vi "Configure Maker Units.vi"(6 "Reset Y Position (T: Enable)":bool=TRUE, 7 "Reset X Position (T: Enable)":bool=TRUE, 8 "error in (no error)":errorcluster, 9 "Marker Y Units (0: Base)":i32(ring) items=["Base", "Percent"], 10 "Marker X Units (0: Seconds)":i32(ring) items=["Seconds", "Hertz", "Degrees", "Percent"], 11 "VISA resource name":refnum<visa-resource-name>) -> (0 "error out":errorcluster, 3 "VISA resource name out":refnum<visa-resource-name>)   [LabVIEW 2016, in "Agilent 2000 3000 X-Series.lvlib"]
doc: "Configures the marker unit settings."
uses:
  Agilent 2000 3000 X-Series.lvlib
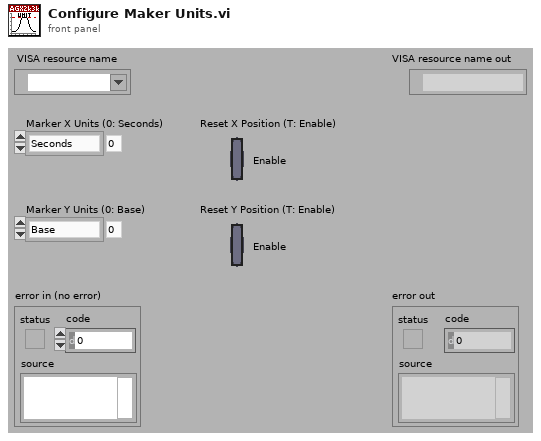
[diagram p1: front panel]
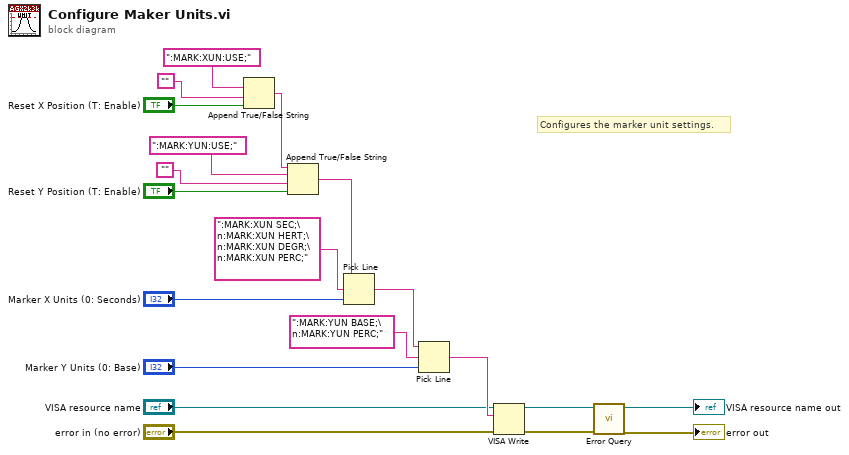
[diagram p0: block diagram]
diagram:
  # "Configures the marker unit settings."
  n1 = Append True/False String(1:"Reset X Position (T: Enable)", 2:"", 3:":MARK:XUN:USE;") -> (0:w6:string)  [unwired: 1 out]
  n2 = Append True/False String(1:"Reset Y Position (T: Enable)", 2:"", 3:":MARK:YUN:USE;", 4:w6) -> (0:w3:string)
  n3 = Pick Line(string ("")=w3, multi-line string=":MARK:XUN SEC;\n:MARK:XUN HERT;\n:MARK:XUN DEGR;\n:MARK:XUN PERC;", line index="Marker X Units (0: Seconds)") -> (output string=w16:string)
  n4 = Pick Line(string ("")=w16, multi-line string=":MARK:YUN BASE;\n:MARK:YUN PERC;", line index="Marker Y Units (0: Base)") -> (output string=w15:string)
  n5 = VISA Write(VISA resource name="VISA resource name", write buffer=w15, error in (no error)="error in (no error)") -> (VISA resource name out=w12:refnum<visa-resource-name>, error out=w11:errorcluster)  [unwired: 1 out]
  n6 = call "Error Query.vi"("error in (no error)"=w11, "VISA resource name"=w12) -> ("error out"=→"error out":errorcluster, "VISA resource name out"=→"VISA resource name out":refnum<visa-resource-name>)  [unwired: 8 out]
